vi "Error Code.vi"(0 "Enable":bool=TRUE, 5 "error in (no error)":errorcluster) -> (14 "Error Code 2":string, 18 "OK":bool, 19 "error out":errorcluster)   [LabVIEW 2017]
doc: "Displays a standard dialog box that prompts users to enter information, such as a user name and password.\n--------------------\n\nThis Express VI is configured as follows:\n\nMessage to Display to the User:\nThe inputs are: \nNumber: c002"
panel:
  in  "Error Code":string(combo)
  in  "Cancel":bool
  in  "OK2":bool
  in  "OK1":bool
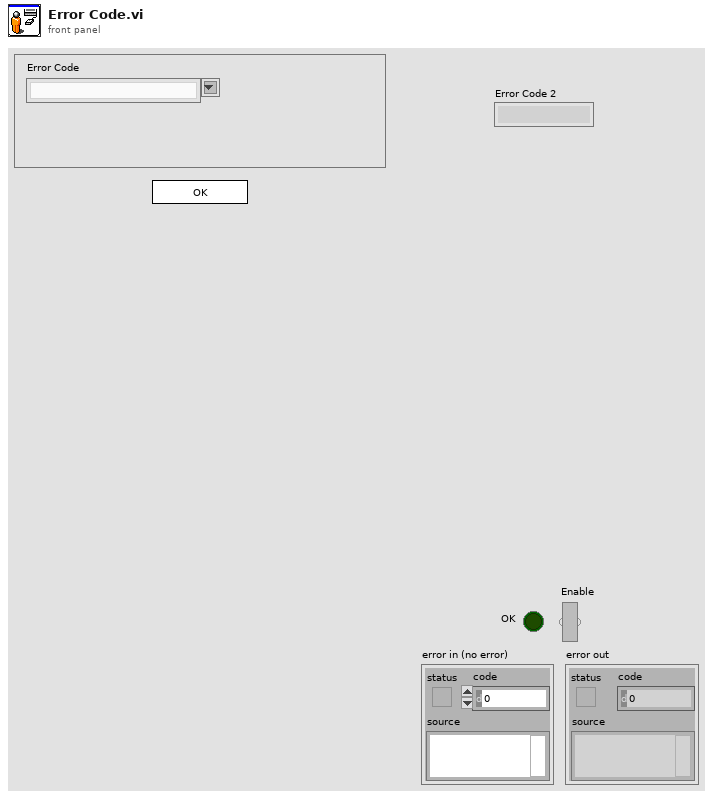
[diagram p1: front panel]
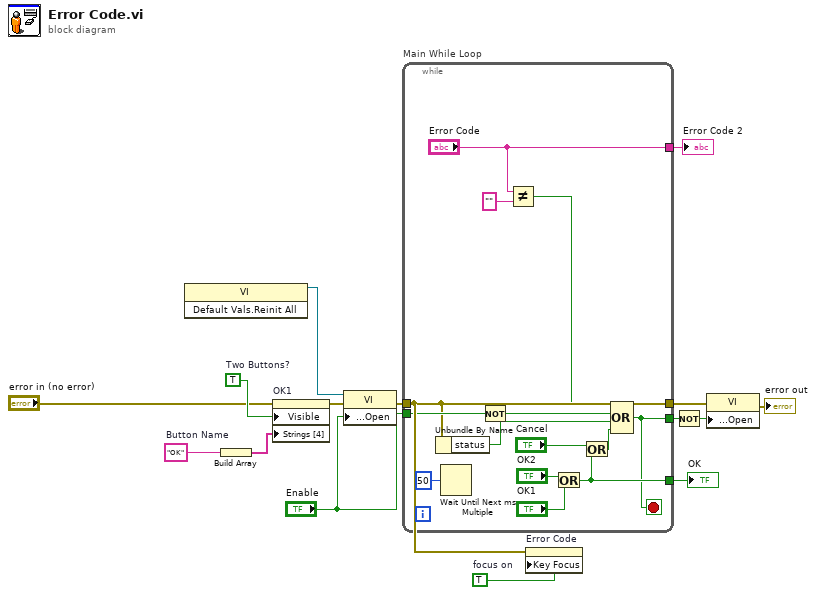
[diagram p0: block diagram]
diagram:
  w2 = TRUE  # focus on
  w10 = "OK"  # Button Name
  w14 = TRUE  # Two Buttons?
  n1 = invoke class="VI" method="Default Vals.Reinit All"() -> (reference out=w3:refnum<vi>)  [unwired: 3 in, 2 out]
  n2 = Build Array(w10) -> (w11:string[])
  n3 = property on="OK1" class="Bool"(error in="error in (no error)", "Visible"=w14, "Strings [4]"=w11) -> (error out=w9:errorcluster)  [unwired: 1 in, 1 out]
  n4 = property class="VI"(reference=w3, error in=w9, "Front Panel Window:Open"="Enable") -> (error out=w8:errorcluster)  [unwired: 1 out]
  n5 = while "Main While Loop" {
    tunnel: [w26] -> w15
    tunnel: "Enable" -> [w24]
    tunnel: [w22] -> w12
    tunnel: w8 -> [w21]
    tunnel: [w21] -> w6
    tunnel: ["Error Code"] -> w1
    stop <- w22 stop-if-true
    n6 = Unbundle By Name(w21) -> ("status"=w19:bool)
    n7 = Wait Until Next ms Multiple(millisecond multiple=u32 50) -> ()  [unwired: 1 out]
    n8 = Not(x=w24) -> (.not. x?=w23:bool)
    n9 = Not Equal?(x="Error Code", y="") -> (x != y?=w16:bool)
    n10 = Or(x="OK2", y="OK1") -> (x .or. y?=w26:bool)
    n11 = Or(x="Cancel", y=w26) -> (x .or. y?=w20:bool)
    n12 = Compound Arithmetic op=OR(w16, w23, w19, w20) -> (w22:bool)
  }
  "OK" <- w15
  "Error Code 2" <- w1
  n13 = property on="Error Code" class="CmbBox"(error in=w8, "Key Focus"=w2) -> ()  [unwired: 1 in, 2 out]
  n14 = Not(x=w12) -> (.not. x?=w13:bool)
  n15 = property class="VI"(error in=w6, "Front Panel Window:Open"=w13) -> (error out=→"error out":errorcluster)  [unwired: 1 in, 1 out]
